vi "Initializer.vi"(8 "error in (no error)":errorcluster, 11 "UDP_Receiver in":refnum<class "UDP_Receiver.lvclass">) -> (0 "error out":errorcluster, 3 "UDP_Receiver out":refnum<class "UDP_Receiver.lvclass">)   [LabVIEW 2021, in "UDP_Receiver.lvclass"]
uses:
  UDP_Receiver.lvclass
  UDP_Comm/UDP_Comm.lvclass
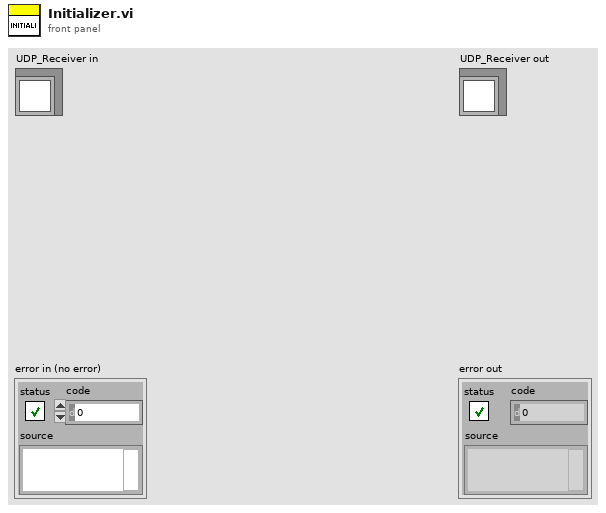
[diagram p1: front panel]
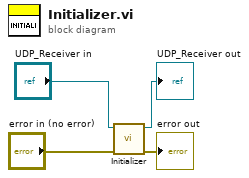
[diagram p0: block diagram]
diagram:
  n1 = call-parent "Initializer.vi"("error in (no error)"="error in (no error)", "UDP_Comm in"="UDP_Receiver in") -> ("error out"=→"error out":errorcluster, "UDP_Comm out"=→"UDP_Receiver out":refnum<class "UDP_Receiver.lvclass">)  [unwired: 8 in]
